vi "FTW_AppLauncher-Core_Config_Parse.vi"(0 "Config String":string, 11 "error in":errorcluster) -> (4 "Actors":string[](array[string]), 6 "Configurations":string[](array[string]), 15 "error out":errorcluster)   [LabVIEW 2013, in "FTW-AppLauncher-Core.lvclass"]
uses:
  FTW-AppLauncher-Core.lvclass
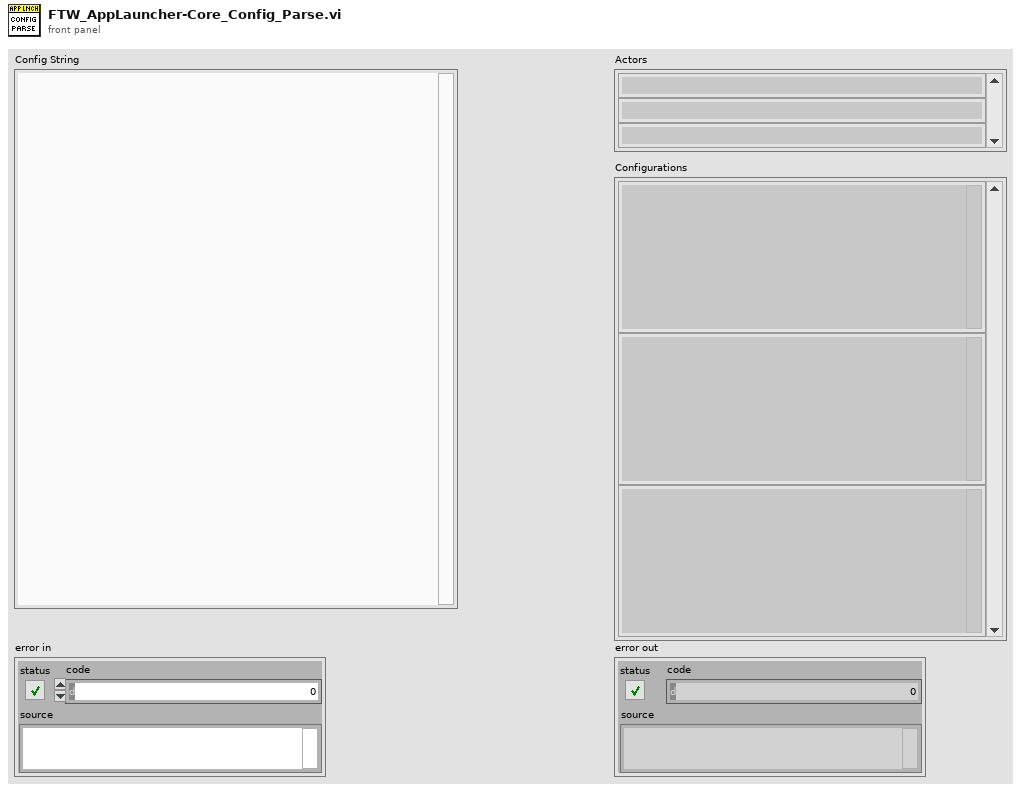
[diagram p1: front panel]
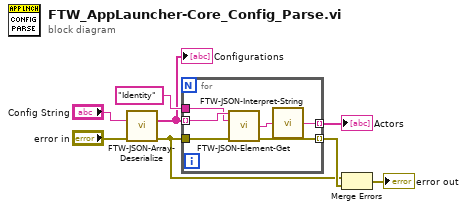
[diagram p0: block diagram]
diagram:
  n1 = call "FTW-JSON-Array-Deserialize.vi"("Array of JSON Objects"="Config String", "error in"="error in") -> ("JSON Elements"=w3:string[], "error out"=w1:errorcluster)  [unwired: 11 in, 1 out]
  "Configurations" <- w3
  n2 = for {
    tunnel: w3 -> [w11] mode=indexing
    tunnel: [w9] -> w2 mode=indexing
    tunnel: "Identity" -> [w10]
    tunnel: w1 -> [w14]
    tunnel: [w13] -> w6 mode=indexing
    n3 = call "FTW-JSON-Element-Get.vi"("JSON Opject"=w11, "Key"=w10, "error in"=w14) -> ("Element"=w12:string, "error out"=w13:errorcluster)  [unwired: 10 in, 1 out]
    n4 = call "FTW-JSON-Interpret-String.vi"("JSON String"=w12) -> ("LabVIEW String"=w9:string)
  }
  "Actors" <- w2
  n5 = Merge Errors(w1, w6) -> (→"error out":errorcluster)
